vi "TH_DataBackup.vi"(4 "error in (no error)":errorcluster, 7 "Backup År":u16(ring) items=["2001", "2002", "2003", "2004", "2005", "2006", "2007", "2008", "2009", "2010"]) -> (0 "error out":errorcluster, 3 "return code":i32)   [LabVIEW 2020]
panel:
  out "CommandLine":string
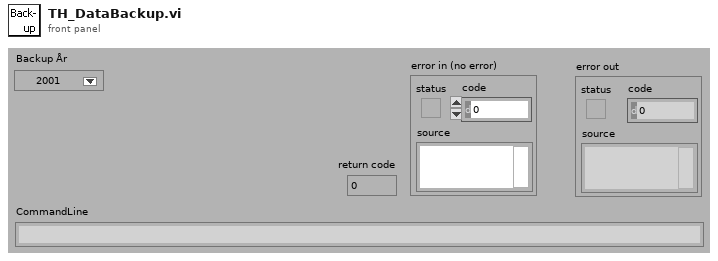
[diagram p1: front panel]
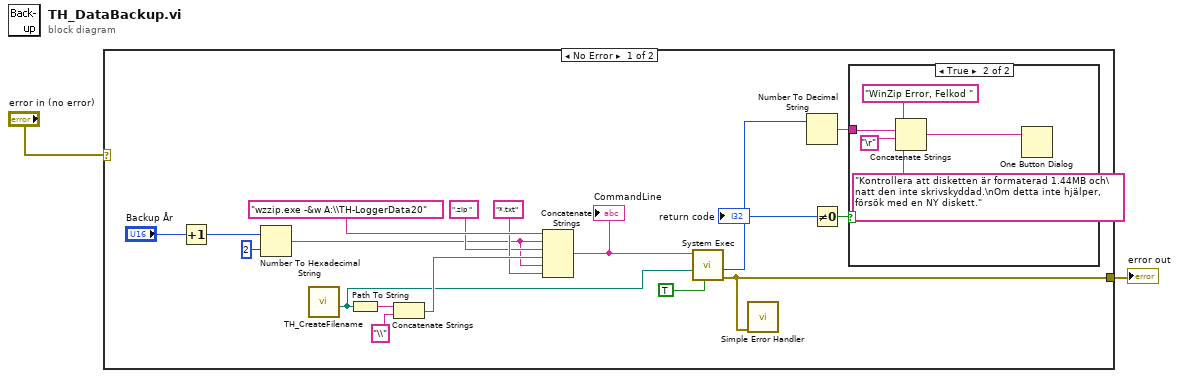
[diagram p0: block diagram]
diagram:
  n1 = case shown="No Error" "error in (no error)" {
    selector: "error in (no error)" -> [_ w25]
    tunnel: [w6 w25] -> w1
    frame No Error {
      n2 = Increment(x="Backup År") -> (x+1=w18:u16)
      n3 = Number To Hexadecimal String(1:i16 2 ("width (-)"), 2:w18) -> (0:w9:string)
      n4 = call "TH_CreateFilename.vi"() -> ("DataPath"=w8:path)  [unwired: 5 in, 2 out]
      n5 = Path To String(path=w8) -> (string=w15:string)
      n6 = Concatenate Strings(w15, "\\") -> (w13:string)
      n7 = Concatenate Strings("wzzip.exe -&w A:\\TH-LoggerData20", w9, ".zip " ("Substring"), w13, w9, "*.txt" ("command line")) -> (w11:string)
      "CommandLine" <- w11
      n8 = call <vilib>:"System Exec.vi"("run minimized? (F)"=TRUE, "working directory"=w8, "command line"=w11) -> ("error out"=w6:errorcluster, "return code"=w4:i32)  [unwired: 5 in, 2 out]
      "return code" <- w4
      n9 = call <vilib>:"Simple Error Handler.vi"("error in (no error)"=w6) -> ()  [unwired: 4 in, 5 out]
      n10 = Number To Decimal String(number=w4) -> (decimal integer string=w3:string)  [unwired: 1 in]
      n11 = Not Equal To 0?(x=w4) -> (x != 0?=w5:bool)
      n12 = case shown="True" w5 {
        tunnel: w3 -> [_ w21]
        frame False {
        }
        frame True {
          n13 = Concatenate Strings("WinZip Error, Felkod ", w21, "\r", "Kontrollera att disketten är formaterad 1.44MB och\natt den inte skrivskyddad.\nOm detta inte hjälper, försök med en NY diskett.") -> (w24:string)
          n14 = One Button Dialog(message=w24) -> ()  [unwired: 1 in, 1 out]
        }
      }
    }
    frame Error {
    }
  }
  "error out" <- w1
